vi "Ballard 429 - Initialize.vi"(7 "RT Config Filepath":path, 8 "Error (in)":errorcluster, 11 "Card Parameters (in)":T1) -> (0 "Error (out)":errorcluster, 3 "Card Parameters (out)":T1)   [LabVIEW 2016, in "Ballard Arinc-429 Engine.lvlib"]
doc: "Arinc-429 Board Initialization."
uses:
  Ballard Arinc-429 Engine.lvlib
  RT Controls/Card Parameters.ctl
  Shared/Controls and Global/Initialization Method.ctl
  <instrlib>/BTICardLib/Private/Initialize By Card Number and Core Number.vi
  <instrlib>/BTICardLib/Private/Initialize By Slot Number and Core Number.vi
  <instrlib>/BTICardLib/Private/IO/Action-Status/Write External LED.vi
  <instrlib>/BTICardLib/Private/Configure All From XML.vi
  <instrlib>/BTI429Lib/Private/Core/Action-Status/Start All Channels.vi
  <instrlib>/BTICardLib/BTICardLV.lvlib
  <instrlib>/BTI429Lib/BTI429LV.lvlib
  Shared/Ballard Arinc-429 Shared.lvlib
  <vilib>/NI VeriStand/Custom Device Tools/Custom Device Utility Library/Custom Device Utility Library.lvlib
panel:
  out "Card Type":string
  out "Product String":string
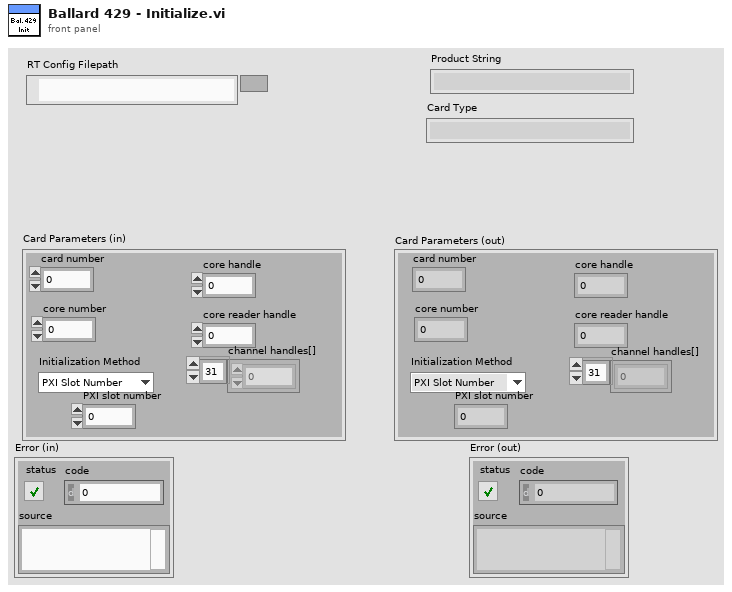
[diagram p1: front panel]
types:
  T1 = typedef "Ballard Arinc-429 Engine.lvlib/Card Parameters.ctl" = cluster{"card number":i32, "core number":i32, "core handle":u64, "core reader handle":u64, "channel handles[]":u64[], "Initialization Method":T2, "PXI slot number":i32}
  T2 = typedef "Ballard Arinc-429 Shared.lvlib/Initialization Method.ctl" = enum16{"PXI Slot Number", "Card Number"}
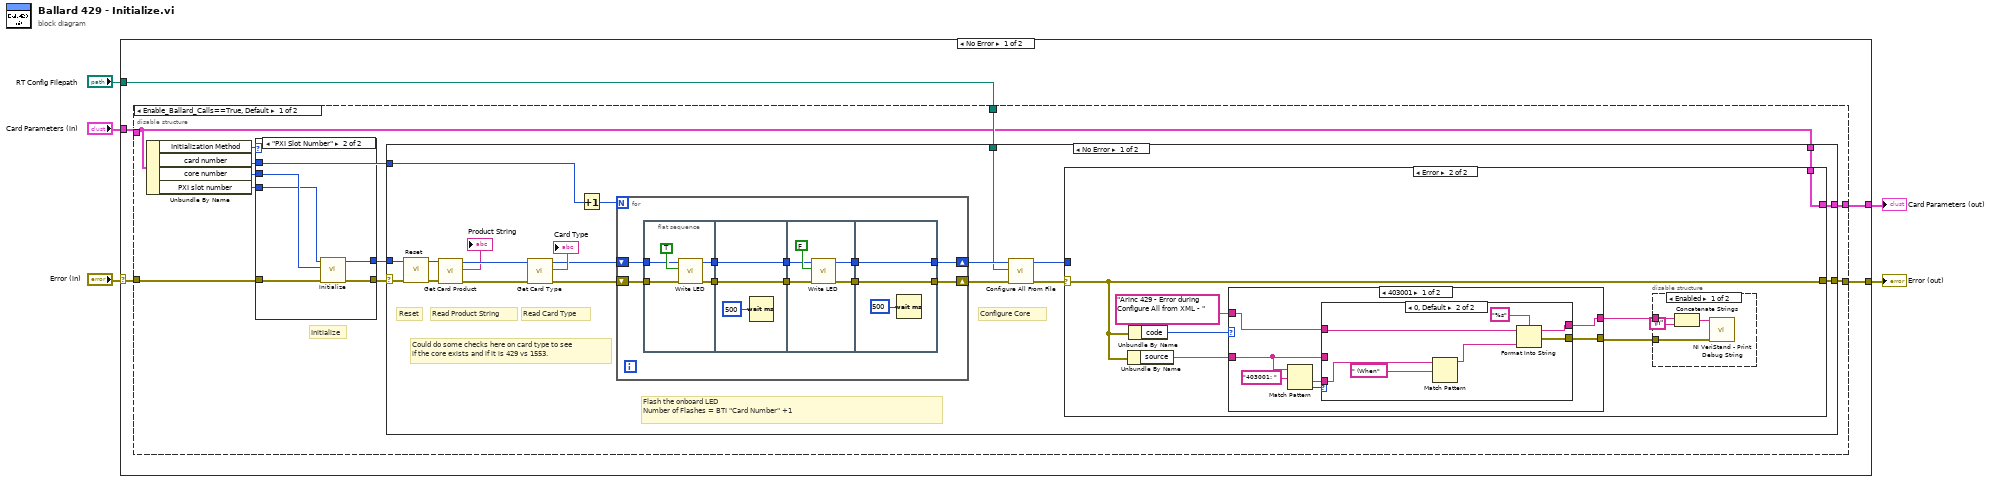
[diagram p0: block diagram]
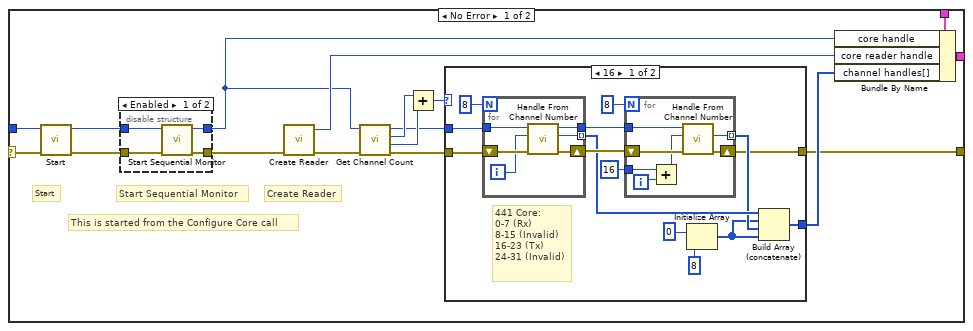
[diagram p2: hidden frame]
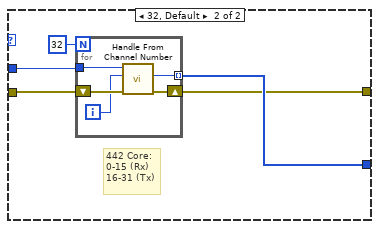
[diagram p3: hidden frame]
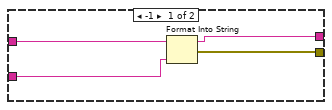
[diagram p6: hidden frame]
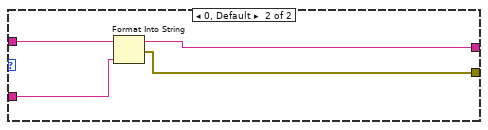
[diagram p7: hidden frame]
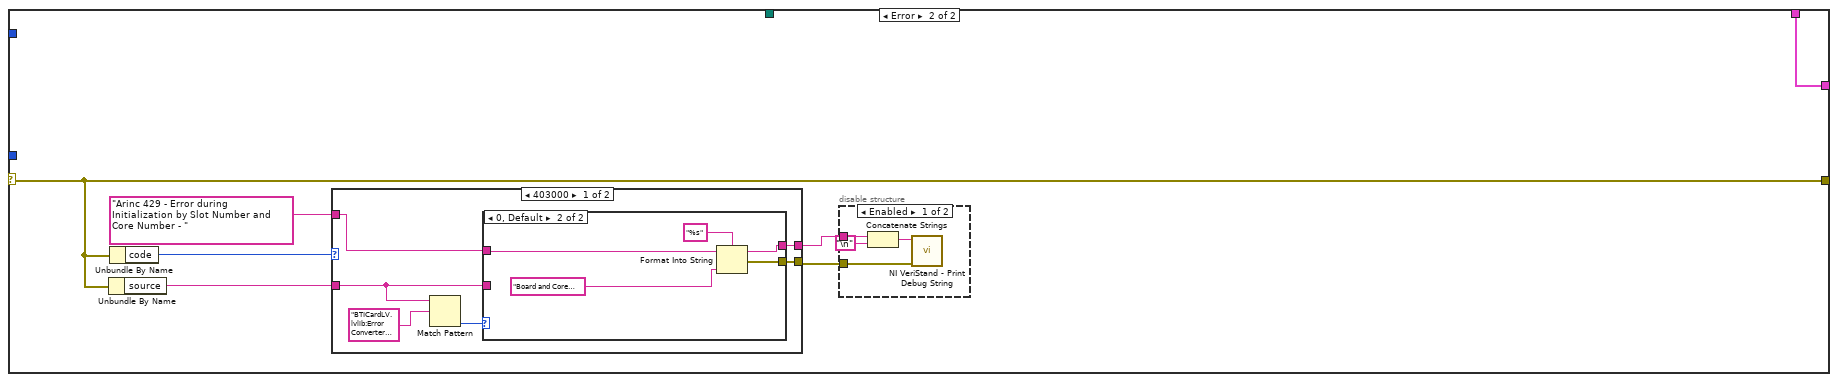
[diagram p8: hidden frame]
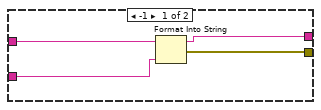
[diagram p10: hidden frame]
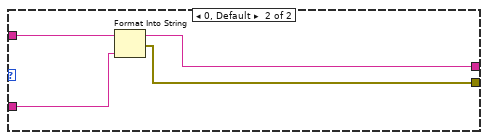
[diagram p11: hidden frame]
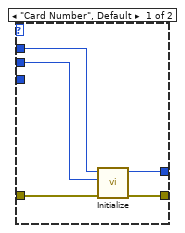
[diagram p12: hidden frame]
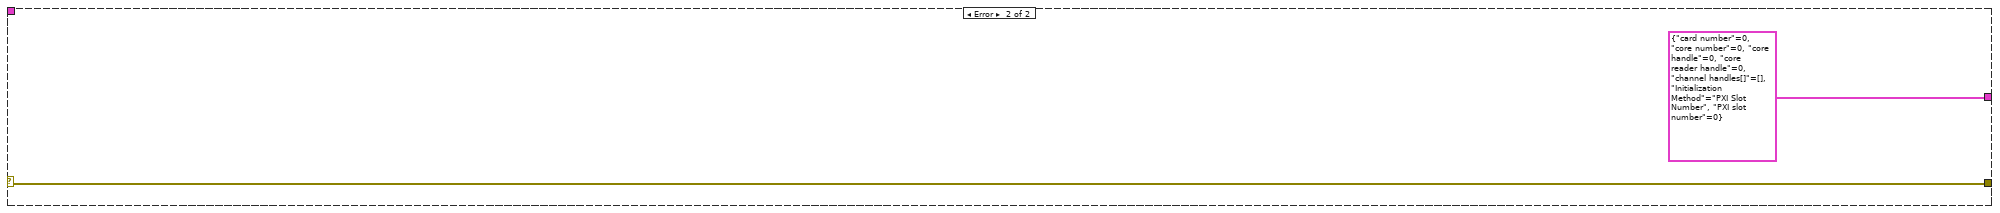
[diagram p14: hidden frame]
diagram:
  n1 = case shown="No Error" "Error (in)" {
    selector: "Error (in)" -> [w7 w204]
    tunnel: [w10 T1 {"card number"=0, "core number"=0, "core handle"=0, "core reader handle"=0, "channel handles[]"=[], "Initialization Method"=enum."PXI Slot Number", "PXI slot number"=0} ("Card Parameters (in)")] -> w5
    tunnel: "RT Config Filepath" -> [w9 _]
    tunnel: [w8 w204] -> w3
    tunnel: "Card Parameters (in)" -> [w6 _]
    frame No Error {
      n2 = disable-structure shown="Enable_Ballard_Calls==True, Default" {
        disable-tunnel: [w20 w201] -> w10
        disable-tunnel: w9 -> [w19 _]
        disable-tunnel: [w12 w202] -> w8
        disable-tunnel: w7 -> [w18 w202]
        disable-tunnel: w6 -> [w17 w201]
        frame condition #0 (active) {
          # "Initialize"
          n3 = Unbundle By Name(w17) -> ("Initialization Method"=w16:T2, "card number"=w15:i32, "core number"=w14:i32, "PXI slot number"=w13:i32)
          n4 = case shown="\"PXI Slot Number\"" w16 {
            tunnel: [w195 w200] -> w21
            tunnel: [w194 w199] -> w11
            tunnel: w15 -> [w193 _]
            tunnel: w18 -> [w192 w198]
            tunnel: w14 -> [w191 w197]
            tunnel: w13 -> [_ w196]
            frame "Card Number", Default {
              n5 = call-poly <instrlib>:"Initialize.vi"("error in (no error)"=w192, "core number"=w191, "card number"=w193) -> ("error out"=w194:errorcluster, "core handle out"=w195:u64)  [unwired: 7 in]
            }
            frame "PXI Slot Number" {
              n6 = call-poly <instrlib>:"Initialize.vi"("error in (no error)"=w198, "core number"=w197, "slot number"=w196) -> ("error out"=w199:errorcluster, "core handle out"=w200:u64)  [unwired: 7 in]
            }
          }
          n7 = case shown="No Error" w11 {
            selector: w11 -> [w23 w164]
            tunnel: w21 -> [w41 _]
            tunnel: [w40 w167] -> w20
            tunnel: w19 -> [w27 _]
            tunnel: w17 -> [w26 w167]
            tunnel: w15 -> [w25 _]
            tunnel: [w24 w164] -> w12
            frame No Error {
              # "Configure Core"
              # "Could do some checks here on card type to see\nif the core exists and if it is 429 vs 1553."
              # "Flash the onboard LED\nNumber of Flashes = BTI \"Card Number\" +1"
              # "Read Card Type"
              # "Read Product String"
              # "Reset"
              n8 = call <instrlib>:"Reset.vi"("error in (no error)"=w23, "core handle in"=w41) -> ("error out"=w34:errorcluster, "core handle out"=w35:u64)  [unwired: 8 in]
              n9 = call <instrlib>:"Get Card Product.vi"("error in (no error)"=w34, "core handle in"=w35) -> ("error out"=w38:errorcluster, "product string out"=→"Product String":string, "core handle out"=w39:u64)  [unwired: 7 in]
              n10 = call <instrlib>:"Get Card Type.vi"("error in (no error)"=w38, "core handle in"=w39) -> ("error out"=w32:errorcluster, "type string out"=→"Card Type":string, "core handle out"=w33:u64)  [unwired: 7 in]
              n11 = Increment(x=w25) -> (x+1=w29:i32)
              n12 = for {
                N: w29 -> [_]
                shift-right: [w136] -> w31
                shift-left: w33 -> [w138]
                shift-right: [w135] -> w30
                shift-left: w32 -> [w137]
                n13 = flat-sequence {
                  tunnel: [w148] -> w144
                  tunnel: [w147] -> w143
                  tunnel: w138 -> [w146]
                  tunnel: w137 -> [w145]
                  tunnel: [w151] -> w142
                  tunnel: w144 -> [w151]
                  tunnel: [w150] -> w141
                  tunnel: w143 -> [w150]
                  tunnel: w142 -> [w156]
                  tunnel: [w155] -> w140
                  tunnel: [w154] -> w139
                  tunnel: w141 -> [w153]
                  tunnel: [w159] -> w135
                  tunnel: w140 -> [w159]
                  tunnel: [w158] -> w136
                  tunnel: w139 -> [w158]
                  frame #0 {
                    n14 = call-poly <instrlib>:"Write LED.vi"("error in (no error)"=w145, "LED state"=TRUE, "core handle in"=w146) -> ("error out"=w148:errorcluster, "core handle out"=w147:u64)  [unwired: 7 in]
                  }
                  frame #1 {
                    n15 = Wait (ms)(milliseconds to wait=u32 500) -> ()  [unwired: 1 out]
                  }
                  frame #2 {
                    n16 = call-poly <instrlib>:"Write LED.vi"("error in (no error)"=w156, "LED state"=FALSE, "core handle in"=w153) -> ("error out"=w155:errorcluster, "core handle out"=w154:u64)  [unwired: 7 in]
                  }
                  frame #3 {
                    n17 = Wait (ms)(milliseconds to wait=u32 500) -> ()  [unwired: 1 out]
                  }
                }
              }
              n18 = call-poly <instrlib>:"Configure All From File.vi"("error in (no error)"=w30, "configuration file path"=w27, "core handle in"=w31) -> ("error out"=w22:errorcluster, "core handle out"=w28:u64)  [unwired: 7 in]
              n19 = case shown="Error" w22 {
                selector: w22 -> [w42 w103]
                tunnel: [w58 w102] -> w40
                tunnel: w28 -> [w56 _]
                tunnel: w26 -> [w52 w102]
                tunnel: [w43 w103] -> w24
                frame No Error {
                  # "This is started from the Configure Core call"
                  # "Start"
                  # "Start Sequential Monitor"
                  # "Create Reader"
                  n20 = call-poly <instrlib>:"Start.vi"("error in (no error)"=w42, "core handle in"=w56) -> ("error out"=w54:errorcluster, "core handle out"=w55:u64)  [unwired: 8 in]
                  n21 = disable-structure shown="Enabled" {
                    disable-tunnel: w55 -> [w99 w101]
                    disable-tunnel: w54 -> [w98 w100]
                    disable-tunnel: [w97 w100] -> w53
                    disable-tunnel: [w96 w101] -> w50
                    frame Enabled {
                      n22 = call <instrlib>:"Start Sequential Monitor.vi"("error in (no error)"=w98, "core handle in"=w99) -> ("error out"=w97:errorcluster, "core handle out"=w96:u64)  [unwired: 8 in]
                    }
                    frame Disabled {
                    }
                  }
                  n23 = call <instrlib>:"Create Reader.vi"("error in (no error)"=w53) -> ("error out"=w51:errorcluster, "core reader handle out"=w57:u64)  [unwired: 9 in]
                  n24 = call <instrlib>:"Get Channel Count.vi"("error in (no error)"=w51, "core handle in"=w50) -> ("error out"=w46:errorcluster, "transmit channel count out"=w49:i32, "receive channel count out"=w48:i32, "core handle out"=w45:u64)  [unwired: 6 in]
                  n25 = Add(x=w48, y=w49) -> (x+y=w47:i32)
                  n26 = case shown="16" w47 {
                    tunnel: w46 -> [w71 w89]
                    tunnel: w45 -> [w70 w88]
                    tunnel: [w63 w87] -> w44
                    tunnel: [w60 w86] -> w43
                    frame 16 {
                      # "441 Core:\n0-7 (Rx)\n8-15 (Invalid)\n16-23 (Tx)\n24-31 (Invalid)"
                      n27 = for {
                        N: 8 -> [_]
                        shift-right: [w82] -> w68
                        shift-left: w71 -> [w85]
                        tunnel: [w83] -> w64 mode=indexing
                        tunnel: w70 -> [w81]
                        tunnel: [w80] -> w67
                        i -> [w84]
                        n28 = call <instrlib>:"Handle From Channel Number.vi"("error in (no error)"=w85, "channel number"=w84, "core handle in"=w81) -> ("error out"=w82:errorcluster, "channel handle out"=w83:u64, "core handle out"=w80:u64)  [unwired: 6 in]
                      }
                      n29 = for {
                        N: 8 -> [_]
                        shift-right: [w77] -> w60
                        shift-left: w68 -> [w79]
                        tunnel: [w78] -> w62 mode=indexing
                        tunnel: w67 -> [w76]
                        tunnel: 16 ("channel handle out") -> [w73]
                        i -> [w74]
                        n30 = Add(x=w73, y=w74) -> (x+y=w75:i32)
                        n31 = call <instrlib>:"Handle From Channel Number.vi"("error in (no error)"=w79, "channel number"=w75, "core handle in"=w76) -> ("error out"=w77:errorcluster, "channel handle out"=w78:u64)  [unwired: 6 in, 1 out]
                      }
                      n32 = Initialize Array(u64 0 ("channel handle out"), 8 ("dimension size")) -> (w61:u64[])
                      n33 = Build Array (concatenate)(w64, w61, w62, w61) -> (w63:u64[])
                    }
                    frame 32, Default {
                      # "442 Core:\n0-15 (Rx)\n16-31 (Tx)"
                      n34 = for {
                        N: 32 -> [_]
                        shift-right: [w92] -> w86
                        shift-left: w89 -> [w95]
                        tunnel: [w93] -> w87 mode=indexing
                        tunnel: w88 -> [w91]
                        i -> [w94]
                        n35 = call <instrlib>:"Handle From Channel Number.vi"("error in (no error)"=w95, "channel number"=w94, "core handle in"=w91) -> ("error out"=w92:errorcluster, "channel handle out"=w93:u64)  [unwired: 6 in, 1 out]
                      }
                    }
                  }
                  n36 = Bundle By Name(cluster=w52, "core handle"=w50, "core reader handle"=w57, "channel handles[]"=w44) -> (w58:T1)
                }
                frame Error {
                  n37 = Unbundle By Name(w103) -> ("source"=w106:string)
                  n38 = Unbundle By Name(w103) -> ("code"=w104:i32)
                  n39 = case shown="403001" w104 {
                    tunnel: [w119 w132] -> w108
                    tunnel: [w118 w131] -> w107
                    tunnel: "Arinc 429 - Error during Configure All from XML - " ("String to write") -> [w116 w134]
                    tunnel: w106 -> [w117 w133]
                    frame 403001 {
                      n40 = Match Pattern(string=w117, regular expression="403001: ") -> (after substring=w113:string, offset past match=w115:i32)  [unwired: 1 in, 2 out]
                      n41 = case shown="0, Default" w115 {
                        tunnel: [w120 w130] -> w119
                        tunnel: [w121 w129] -> w118
                        tunnel: w117 -> [w122 _]
                        tunnel: w116 -> [w123 w128]
                        tunnel: w113 -> [_ w126]
                        frame -1 {
                          n42 = Format Into String(initial string=w123, w122) -> (resulting string=w120:string, error out=w121:errorcluster)  [unwired: 2 in]
                        }
                        frame 0, Default {
                          n43 = Match Pattern(string=w126, regular expression=" (When") -> (before substring=w125:string)  [unwired: 1 in, 3 out]
                          n44 = Format Into String(format string="%s", initial string=w128, w125) -> (resulting string=w130:string, error out=w129:errorcluster)  [unwired: 1 in]
                        }
                      }
                    }
                    frame 0, Default {
                      n45 = Format Into String(initial string=w134, w133) -> (resulting string=w132:string, error out=w131:errorcluster)  [unwired: 2 in]
                    }
                  }
                  n46 = disable-structure shown="Enabled" {
                    disable-tunnel: w107 -> [w110 _]
                    disable-tunnel: w108 -> [w109 _]
                    frame Enabled {
                      n47 = Concatenate Strings(w109, "\n") -> (w111:string)
                      n48 = call <vilib>:"NI VeriStand - Print Debug String.vi"("error in (no error)"=w110, "Message"=w111) -> ()  [unwired: 9 in, 1 out]
                    }
                    frame Disabled {
                    }
                  }
                }
              }
            }
            frame Error {
              n49 = Unbundle By Name(w164) -> ("source"=w163:string)
              n50 = Unbundle By Name(w164) -> ("code"=w166:i32)
              n51 = case shown="403000" w166 {
                tunnel: [w177 w188] -> w161
                tunnel: [w176 w187] -> w162
                tunnel: "Arinc 429 - Error during Initialization by Slot Number and Core Number - " ("String to write") -> [w172 w190]
                tunnel: w163 -> [w173 w189]
                frame 403000 {
                  n52 = Match Pattern(string=w173, regular expression="BTICardLV.lvlib:Error Converter (ErrCode or Status).vi<ERR>\nEncountered library error 403000=ERRTYPE_INITIALIZE Failed to initialize the card or core (LabVIEW Library)\nDebug Info: No matching slot number was found in BTICardLV_InitializeBySlotNumber.") -> (offset past match=w174:i32)  [unwired: 1 in, 3 out]
                  n53 = case shown="0, Default" w174 {
                    tunnel: [w178 w186] -> w177
                    tunnel: [w179 w185] -> w176
                    tunnel: w173 -> [w180 _]
                    tunnel: w172 -> [w181 w184]
                    frame -1 {
                      n54 = Format Into String(initial string=w181, w180) -> (resulting string=w178:string, error out=w179:errorcluster)  [unwired: 2 in]
                    }
                    frame 0, Default {
                      n55 = Format Into String(format string="%s", initial string=w184, "Board and Core combination cannot be found. Ensure Initialization method and parameters values are valid.") -> (resulting string=w186:string, error out=w185:errorcluster)  [unwired: 1 in]
                    }
                  }
                }
                frame 0, Default {
                  n56 = Format Into String(initial string=w190, w189) -> (resulting string=w188:string, error out=w187:errorcluster)  [unwired: 2 in]
                }
              }
              n57 = disable-structure shown="Enabled" {
                disable-tunnel: w162 -> [w169 _]
                disable-tunnel: w161 -> [w168 _]
                frame Enabled {
                  n58 = Concatenate Strings(w168, "\n") -> (w170:string)
                  n59 = call <vilib>:"NI VeriStand - Print Debug String.vi"("error in (no error)"=w169, "Message"=w170) -> ()  [unwired: 9 in, 1 out]
                }
                frame Disabled {
                }
              }
            }
          }
        }
        frame condition #1 {
        }
      }
    }
    frame Error {
    }
  }
  "Error (out)" <- w3
  "Card Parameters (out)" <- w5
